vi "ArduinoFinal.vi"(8 "Error In":errorcluster, 10 "Knob":u8(knob)=4 scale=4.0..10.0, 11 "Serial Port":refnum<visa-resource-name>="COM4") -> (0 "Error Out":errorcluster, 2 "Response":u8[](array[numeric]))   [LabVIEW 2015]
uses:
  <vilib>/MakerHub/LINX/Public/Utilities/Open Serial.vi
  <vilib>/MakerHub/LINX/LMH-LINX.lvlib
panel:
  in  "?":bool
  out "Input Array":u8[](array[numeric])
  out "Delay (Hz)":u32
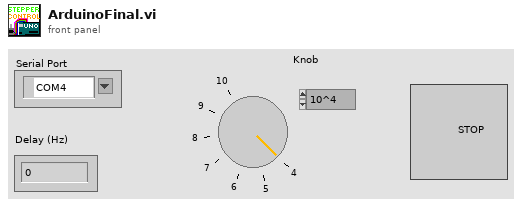
[diagram p1: front panel]
types:
  T1 = typedef "LMH-LINX.lvlib/LINX Ref.ctl" = cluster{"IO":T2, "Interface":T3, "LINX Device Config":T4}
  T2 = typedef "LMH-LINX.lvlib/Platform.ctl" = enum16{"Remote", "Local"}
  T3 = typedef "LMH-LINX.lvlib/Interface.ctl" = enum16{"Serial", "TCP"}
  T4 = typedef "LMH-LINX.lvlib/Device.lvlib/LINX Device Config.ctl" = cluster{"Interface":T3, "COM Port":refnum<visa-resource-name>, "TCP Configuration":T5, "Device Family":u8, "Device ID":u8, "Device Name":string, "TCP Ref":refnum<k5>, "Channels":T6}
  T5 = typedef "LMH-LINX.lvlib/Device.lvlib/TCP Config.ctl" = cluster{"IP Address":string, "Port":u16}
  T6 = typedef "LMH-LINX.lvlib/Channels.ctl" = cluster{"DI":u8[], "DO":u8[], "AI":u8[], "AO":u8[], "PWM":u8[], "QE":u8[], "UART":u8[], "I2C 2":u8[], "SPI":u8[], "CAN":u8[], "Servo":u8[], "AI Ref (V)":dbl, "AI Resolution (Bits)":u8, "AO Ref (V)":dbl, "AO Resolution (Bits)":u8}
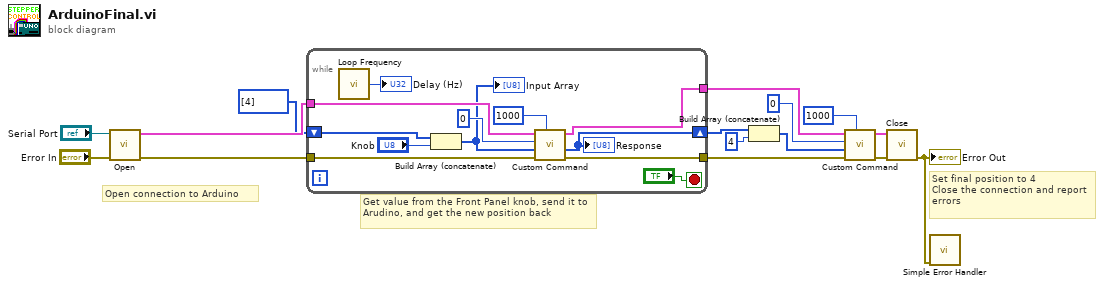
[diagram p0: block diagram]
diagram:
  # "Set final position to 4\nClose the connection and report errors"
  # "Get value from the Front Panel knob, send it to Arudino, and get the new position back"
  # "Open connection to Arduino"
  n1 = call-poly <vilib>:"Open.vi"("Error In"="Error In", "Serial Port"="Serial Port") -> ("Error Out"=w13:errorcluster, "LINX Resource"=w14:T1)  [unwired: 7 in, 1 out]
  n2 = while {
    tunnel: w14 -> [w24]
    tunnel: [w27] -> w10
    tunnel: [w25] -> w9
    tunnel: w13 -> [w26]
    shift-right: [w23] -> w2
    shift-left: u8[] [4] ("Response") -> [w22]
    stop <- "?" stop-if-true
    n3 = call <vilib>:"Loop Frequency.vi"() -> ("Loop Rate (Hz)"=→"Delay (Hz)":u32)
    n4 = Build Array (concatenate)(w22, "Knob") -> (w19:u8[])
    "Input Array" <- w19
    n5 = call <vilib>:"Custom Command.vi"("Timeout (100 ms)"=1000, "Error In"=w26, "Data"=w19, "Custom Command Number"=u16 0, "LINX Resource"=w24) -> ("Error Out"=w25:errorcluster, "Response"=w23:u8[], "LINX Resource"=w27:T1)  [unwired: 3 in, 1 out]
    "Response" <- w23
  }
  n6 = Build Array (concatenate)(w2, u8 4) -> (w5:u8[])
  n7 = call <vilib>:"Custom Command.vi"("Timeout (100 ms)"=1000, "Error In"=w9, "Data"=w5, "Custom Command Number"=u16 0, "LINX Resource"=w10) -> ("Error Out"=w8:errorcluster, "LINX Resource"=w7:T1)  [unwired: 3 in, 2 out]
  n8 = call <vilib>:"Close.vi"("Error In"=w8, "LINX Resource"=w7) -> ("Error Out"=w11:errorcluster)  [unwired: 9 in]
  "Error Out" <- w11
  n9 = call <vilib>:"Simple Error Handler.vi"("error in (no error)"=w11) -> ()  [unwired: 4 in, 5 out]
